vi "Percent Complete Global.vi"() -> ()   [LabVIEW 2025]
panel:
  in  "Percent Complete":dbl
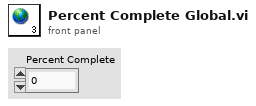
[diagram p1: front panel]
diagram:
